vi "vazão do ar(SubVI).vi"(11 "data in":string) -> (3 "Numeric":dbl)   [LabVIEW 2015]
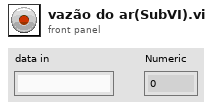
[diagram p1: front panel]
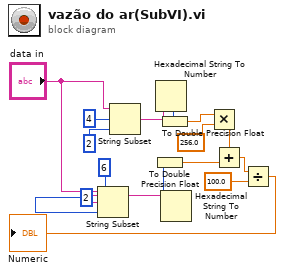
[diagram p0: block diagram]
diagram:
  n1 = String Subset(string="data in", offset (0)=6, length (rest)=2 ("length (rest)")) -> (substring=w14:string)
  n2 = String Subset(string="data in", offset (0)=4, length (rest)=2 ("length (rest)")) -> (substring=w3:string)
  n3 = Hexadecimal String To Number(string=w3) -> (number=w5:u32)  [unwired: 2 in, 1 out]
  n4 = To Double Precision Float(number=w5) -> (double precision float=w11:dbl)
  n5 = Hexadecimal String To Number(string=w14) -> (number=w4:u32)  [unwired: 2 in, 1 out]
  n6 = To Double Precision Float(number=w4) -> (double precision float=w12:dbl)
  n7 = Multiply(x=w11, y=256.0) -> (x*y=w13:dbl)
  n8 = Add(x=w13, y=w12) -> (x+y=w9:dbl)
  n9 = Divide(x=w9, y=100.0) -> (x/y=→"Numeric":dbl)
